vi "Figure Window.vi"(4 "Y scale label (amplitude (V))":string="amplitude (V)", 5 "Data name (samples)":string="samples", 6 "X scale label (time(s))":string="time (s)", 7 "Plot name (sampled signal)":string="Sampled signal", 11 "data qeue":refnum<queue>) -> ()   [LabVIEW 2020]
uses:
  <vilib>/Utility/error.llb/Error Cluster From Error Code.vi
  <vilib>/ErrorRing/Error Ring.xnode
  external libraries/varilib/varilib.lvlib
panel:
  out "external called for stop":bool
  out "title":string
  in  "Keep opened":bool=TRUE
  out "XY Graph":cluster{dbl[], dbl[]}(graph)
  in  "rectangle zoom":bool
  in  "zoom out":bool
  in  "y zoom":bool
  in  "x zoom":bool
  out "gui_elements":refnum<vi>[](array[refnum])
  in  "cancel":bool
  in  "export to excell":bool
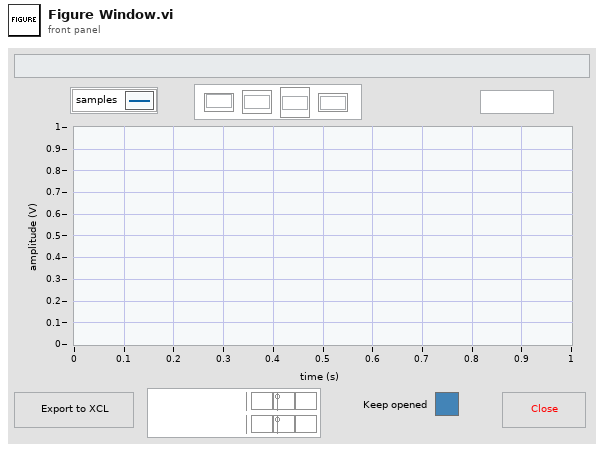
[diagram p1: front panel]
types:
  T1 = typedef "LVRectTypeDef.ctl" = cluster{"Left":i16, "Top":i16, "Right":i16, "Bottom":i16}
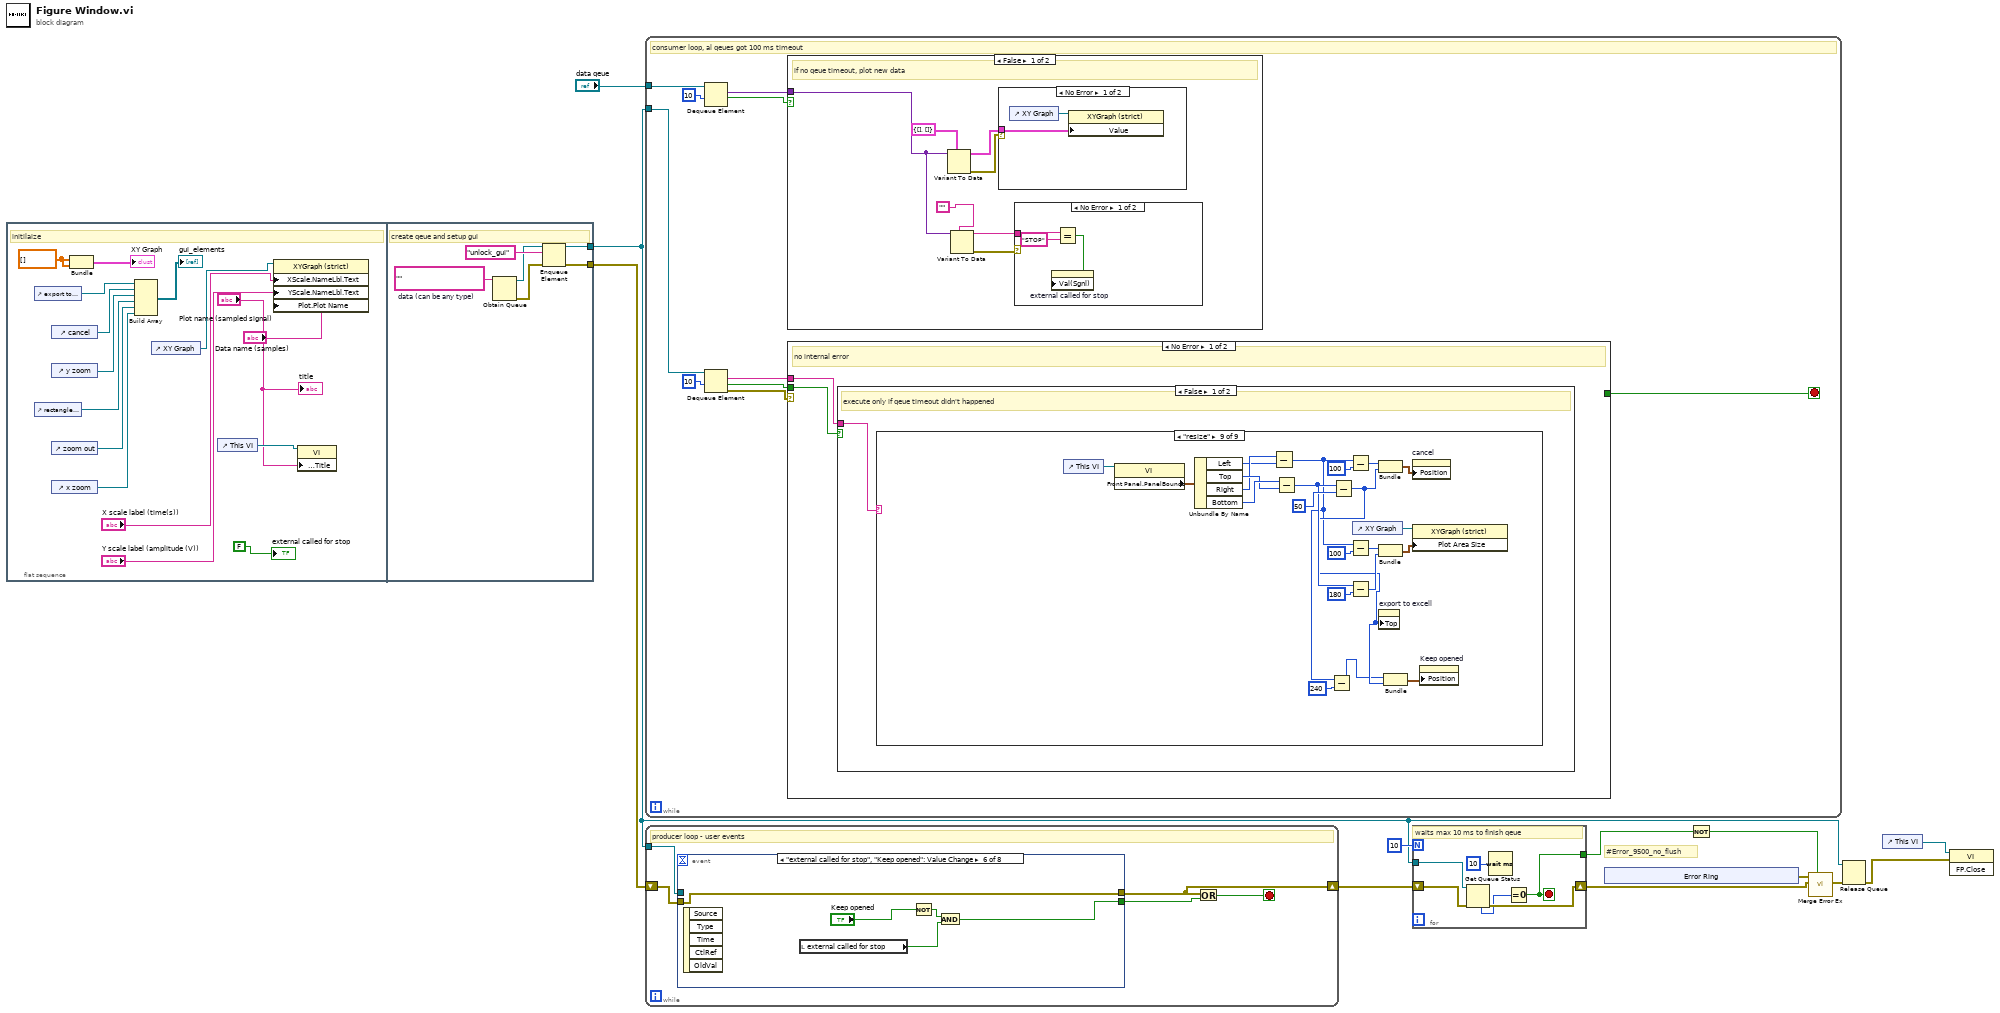
[diagram p0: block diagram]
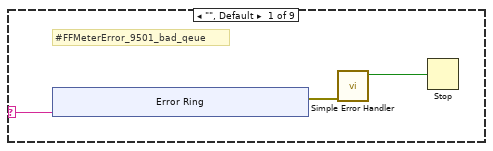
[diagram p5: hidden frame]
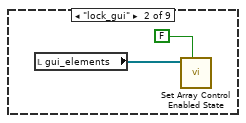
[diagram p6: hidden frame]
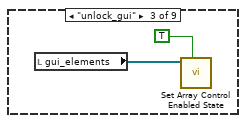
[diagram p7: hidden frame]
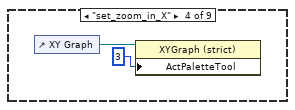
[diagram p8: hidden frame]
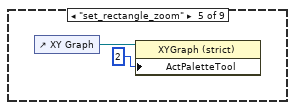
[diagram p9: hidden frame]
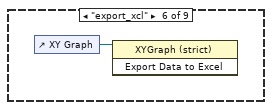
[diagram p10: hidden frame]
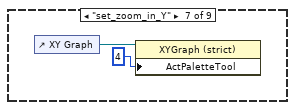
[diagram p11: hidden frame]
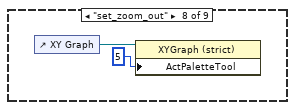
[diagram p12: hidden frame]
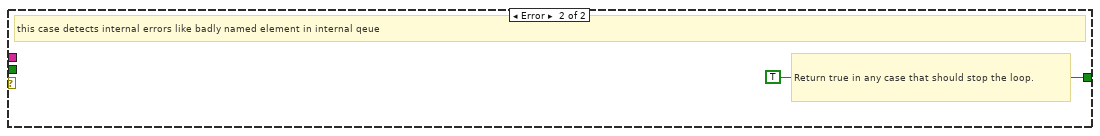
[diagram p14: hidden frame]
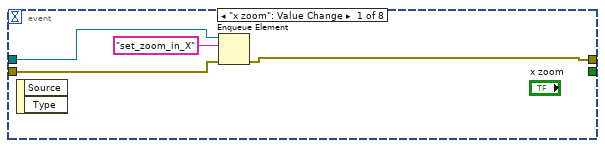
[diagram p15: hidden frame]
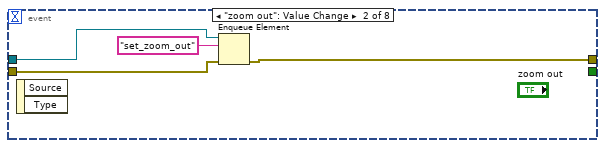
[diagram p16: hidden frame]
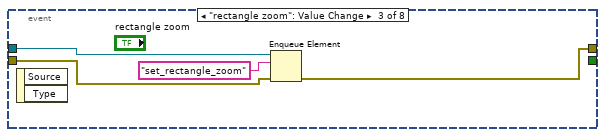
[diagram p17: hidden frame]
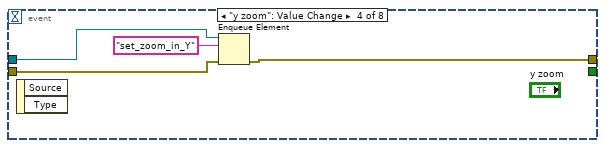
[diagram p18: hidden frame]
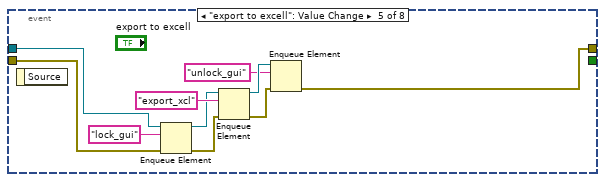
[diagram p19: hidden frame]
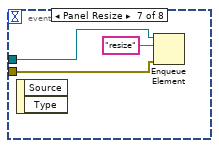
[diagram p20: hidden frame]
diagram:
  # "#Error_9500_no_flush"
  n1 = flat-sequence {
    tunnel: [w33] -> w5
    tunnel: [w31] -> w4
    frame #0 {
      w20 = dbl[] []
      # "initilaize"
      n2 = control-ref of="export to excell"() -> (w28:refnum<vi>)
      n3 = control-ref of="rectangle zoom"() -> (w24:refnum<vi>)
      n4 = control-ref of="cancel"() -> (w27:refnum<vi>)
      n5 = control-ref of="y zoom"() -> (w25:refnum<vi>)
      n6 = control-ref of="zoom out"() -> (w23:refnum<vi>)
      n7 = control-ref of="x zoom"() -> (w22:refnum<vi>)
      n8 = Bundle(w20, w20) -> (→"XY Graph":cluster{dbl[], dbl[]})  [unwired: 1 in]
      n9 = Build Array(w28, w27, w25, w24, w23, w22) -> (→"gui_elements":refnum<vi>[])
      n10 = control-ref of="XY Graph"() -> (w19:refnum<vi>)
      n11 = control-ref of="This VI"() -> (w16:refnum<vi>)
      n12 = property class="XYGraph (strict)"(reference=w19, "XScale.NameLbl.Text"="X scale label (time(s))", "YScale.NameLbl.Text"="Y scale label (amplitude (V))", "Plot.Plot Name"="Data name (samples)") -> ()  [unwired: 1 in, 2 out]
      n13 = property class="VI"(reference=w16, "Front Panel.Title"="Plot name (sampled signal)") -> ()  [unwired: 1 in, 2 out]
      "title" <- "Plot name (sampled signal)"
      "external called for stop" <- FALSE ("external called for stop")
    }
    frame #1 {
      w32 = ""  # data (can be any type)
      # "create qeue and setup gui"
      n14 = Obtain Queue(element data type=w32) -> (queue out=w30:refnum<queue>, error out=w29:errorcluster)  [unwired: 4 in, 1 out]
      n15 = Enqueue Element(queue=w30, element="unlock_gui", error in (no error)=w29) -> (queue out=w33:refnum<queue>, error out=w31:errorcluster)  [unwired: 1 in, 1 out]
    }
  }
  n16 = while {
    tunnel: w5 -> [w44]
    tunnel: "data qeue" -> [w37]
    stop <- w41 stop-if-true
    # "consumer loop, al qeues got 100 ms timeout"
    n17 = Dequeue Element(queue=w37, timeout in ms (-1)=10) -> (element=w38:variant, timed out?=w39:bool)  [unwired: 1 in, 2 out]
    n18 = Dequeue Element(queue=w44, timeout in ms (-1)=10) -> (element=w42:string, timed out?=w35:bool, error out=w43:errorcluster)  [unwired: 1 in, 1 out]
    n19 = case shown="False" w39 {
      tunnel: w38 -> [w47 _]
      frame False {
        # "if no qeue timeout, plot new data"
        n20 = Variant To Data(type=cluster{dbl[], dbl[]} {[], []} ("output cluster"), Variant=w47) -> (data=w50:cluster{dbl[], dbl[]}, error out=w49:errorcluster)  [unwired: 1 in]
        n21 = Variant To Data(type="", Variant=w47) -> (data=w45:string, error out=w46:errorcluster)  [unwired: 1 in]
        n22 = case shown="No Error" w49 {
          tunnel: w50 -> [w56 _]
          frame No Error {
            n23 = control-ref of="XY Graph"() -> (w55:refnum<vi>)
            n24 = property class="XYGraph (strict)"(reference=w55, "Value"=w56) -> ()  [unwired: 1 in, 2 out]
          }
          frame Error {
          }
        }
        n25 = case shown="No Error" w46 {
          tunnel: w45 -> [w54 _]
          frame No Error {
            n26 = Equal?(x=w54, y="STOP") -> (x = y?=w52:bool)
            n27 = property on="external called for stop" class="Bool (strict)"("Val(Sgnl)"=w52) -> ()  [unwired: 2 in, 2 out]
          }
          frame Error {
          }
        }
      }
      frame True {
      }
    }
    n28 = case shown="No Error" w43 {
      tunnel: w42 -> [w58 _]
      tunnel: [_ TRUE] -> w41
      tunnel: w35 -> [w57 _]
      frame No Error {
        # "no internal error"
        n29 = case shown="False" w57 {
          tunnel: w58 -> [w59 _]
          frame False {
            # "execute only if qeue timeout didn't happened"
            n30 = case shown="\"resize\"" w59 {
              selector: w59 -> [w60 _ _ _ _ _ _ _ _]
              frame "", Default {
                # "#FFMeterError_9501_bad_qeue"
                n31 = xnode "Error Ring"("parameter 0"=w60) -> ("error out"=w62:errorcluster)
                n32 = call <vilib>:"Simple Error Handler.vi"("error in (no error)"=w62) -> ("error?"=w61:bool)  [unwired: 4 in, 4 out]
                n33 = Stop(stop? (T)=w61) -> ()
              }
              frame "lock_gui" {
                n34 = local read "gui_elements"() -> (w71:refnum<vi>[])
                n35 = call "Set Array Control Enabled State.vi"("enabled (T)"=FALSE, "reference array in"=w71) -> ()  [unwired: 8 in, 2 out]
              }
              frame "unlock_gui" {
                n36 = local read "gui_elements"() -> (w73:refnum<vi>[])
                n37 = call "Set Array Control Enabled State.vi"("enabled (T)"=TRUE, "reference array in"=w73) -> ()  [unwired: 8 in, 2 out]
              }
              frame "set_zoom_in_X" {
                n38 = control-ref of="XY Graph"() -> (w74:refnum<vi>)
                n39 = property class="XYGraph (strict)"(reference=w74, "ActPaletteTool"=3 ("Palette:Active Tool")) -> ()  [unwired: 1 in, 2 out]
              }
              frame "set_rectangle_zoom" {
                n40 = control-ref of="XY Graph"() -> (w76:refnum<vi>)
                n41 = property class="XYGraph (strict)"(reference=w76, "ActPaletteTool"=2 ("Palette:Active Tool")) -> ()  [unwired: 1 in, 2 out]
              }
              frame "export_xcl" {
                n42 = control-ref of="XY Graph"() -> (w78:refnum<vi>)
                n43 = invoke class="XYGraph (strict)" method="Export Data to Excel"(reference=w78) -> ()  [unwired: 2 in, 3 out]
              }
              frame "set_zoom_in_Y" {
                n44 = control-ref of="XY Graph"() -> (w79:refnum<vi>)
                n45 = property class="XYGraph (strict)"(reference=w79, "ActPaletteTool"=4 ("Palette:Active Tool")) -> ()  [unwired: 1 in, 2 out]
              }
              frame "set_zoom_out" {
                n46 = control-ref of="XY Graph"() -> (w81:refnum<vi>)
                n47 = property class="XYGraph (strict)"(reference=w81, "ActPaletteTool"=5 ("Palette:Active Tool")) -> ()  [unwired: 1 in, 2 out]
              }
              frame "resize" {
                n48 = control-ref of="This VI"() -> (w90:refnum<vi>)
                n49 = property class="VI"(reference=w90) -> ("Front Panel.PanelBounds"=w91:T1)  [unwired: 1 in, 2 out]
                n50 = Unbundle By Name(w91) -> ("Left"=w92:i16, "Top"=w95:i16, "Right"=w93:i16, "Bottom"=w96:i16)
                n51 = Subtract(x=w93, y=w92) -> (x-y=w83:i16)
                n52 = Subtract(x=w96, y=w95) -> (x-y=w94:i16)
                n53 = Subtract(x=w83, y=i16 240) -> (x-y=w84:i16)
                n54 = Subtract(x=w94, y=i16 50) -> (x-y=w86:i16)
                n55 = Subtract(x=w83, y=i16 100) -> (x-y=w103:i16)
                n56 = Subtract(x=w83, y=i16 100) -> (x-y=w98:i16)
                n57 = Subtract(x=w94, y=i16 180) -> (x-y=w97:i16)
                n58 = control-ref of="XY Graph"() -> (w88:refnum<vi>)
                n59 = Bundle(w103, w86) -> (w104:cluster{i16, i16})  [unwired: 1 in]
                n60 = Bundle(w98, w97) -> (w89:cluster{i16, i16})  [unwired: 1 in]
                n61 = property on="export to excell" class="Bool"("Top"=w86) -> ()  [unwired: 2 in, 2 out]
                n62 = Bundle(w84, w86) -> (w87:cluster{i16, i16})  [unwired: 1 in]
                n63 = property on="cancel" class="Bool"("Position"=w104) -> ()  [unwired: 2 in, 2 out]
                n64 = property class="XYGraph (strict)"(reference=w88, "Plot Area Size"=w89) -> ()  [unwired: 1 in, 2 out]
                n65 = property on="Keep opened" class="Bool (strict)"("Position"=w87) -> ()  [unwired: 2 in, 2 out]
              }
            }
          }
          frame True {
          }
        }
      }
      frame Error {
        # "Return true in any case that should stop the loop."
        # "this case detects internal errors like badly named element in internal qeue"
      }
    }
  }
  n66 = while {
    shift-right: [w106] -> w8
    shift-left: w4 -> [w109]
    tunnel: w5 -> [w110]
    stop <- w107 stop-if-true
    # "producer loop - user events"
    n67 = event shown="[5] \"external called for stop\", \"Keep opened\": Value Change" {
      selector: _ -> [_ _ _ _ _ _ _ _]
      dyn-events: _ -> [_ _ _ _ _ _ _ _]
      timeout: _ -> [_ _ _ _ _ _ _ _]
      tunnel: w110 -> [w111 w115 w119 w123 w134 _ w143 _]
      tunnel: w109 -> [w112 w116 w120 w124 w133 w141 w142 w146]
      tunnel: [w113 w117 w121 w125 w127 w141 _ w146] -> w106
      tunnel: [_ _ _ _ _ w139 _ TRUE ("cancel")] -> w108
      event "x zoom": Value Change {
        n68 = event-data() -> ()  [unwired: 1 in, 2 out]
        n69 = Enqueue Element(queue=w111, element="set_zoom_in_X", error in (no error)=w112) -> (error out=w113:errorcluster)  [unwired: 1 in, 2 out]
      }
      event "zoom out": Value Change {
        n70 = event-data() -> ()  [unwired: 1 in, 2 out]
        n71 = Enqueue Element(queue=w115, element="set_zoom_out", error in (no error)=w116) -> (error out=w117:errorcluster)  [unwired: 1 in, 2 out]
      }
      event "rectangle zoom": Value Change {
        n72 = event-data() -> ()  [unwired: 1 in, 2 out]
        n73 = Enqueue Element(queue=w119, element="set_rectangle_zoom", error in (no error)=w120) -> (error out=w121:errorcluster)  [unwired: 1 in, 2 out]
      }
      event "y zoom": Value Change {
        n74 = event-data() -> ()  [unwired: 1 in, 2 out]
        n75 = Enqueue Element(queue=w123, element="set_zoom_in_Y", error in (no error)=w124) -> (error out=w125:errorcluster)  [unwired: 1 in, 2 out]
      }
      event "export to excell": Value Change {
        n76 = event-data() -> ()  [unwired: 1 in, 1 out]
        n77 = Enqueue Element(queue=w134, element="lock_gui", error in (no error)=w133) -> (queue out=w131:refnum<queue>, error out=w132:errorcluster)  [unwired: 1 in, 1 out]
        n78 = Enqueue Element(queue=w131, element="export_xcl", error in (no error)=w132) -> (queue out=w130:refnum<queue>, error out=w129:errorcluster)  [unwired: 1 in, 1 out]
        n79 = Enqueue Element(queue=w130, element="unlock_gui", error in (no error)=w129) -> (error out=w127:errorcluster)  [unwired: 1 in, 2 out]
      }
      event "external called for stop", "Keep opened": Value Change {
        n80 = event-data() -> ()  [unwired: 1 in, 5 out]
        n81 = local read "external called for stop"() -> (w140:bool)
        n82 = Not(x="Keep opened") -> (.not. x?=w138:bool)
        n83 = And(x=w138, y=w140) -> (x .and. y?=w139:bool)
      }
      event Panel Resize {
        n84 = event-data() -> ()  [unwired: 1 in, 2 out]
        n85 = Enqueue Element(queue=w143, element="resize", error in (no error)=w142) -> ()  [unwired: 1 in, 3 out]
      }
      event "cancel": Value Change; Panel Close {
        n86 = event-data() -> ()  [unwired: 1 in, 2 out]
      }
    }
    n87 = Or(x=w106, y=w108) -> (x .or. y?=w107:bool)
  }
  n88 = for {
    N: 10 -> [_]
    tunnel: w5 -> [w152]
    shift-right: [w150] -> w9
    shift-left: w8 -> [w151]
    tunnel: [w147] -> w6
    stop <- w147 stop-if-true
    # "waits max 10 ms to finish qeue"
    n89 = Get Queue Status(queue=w152, error in (no error)=w151) -> (error out=w150:errorcluster, # elements in queue=w148:i32)  [unwired: 1 in, 6 out]
    n90 = Wait (ms)(milliseconds to wait=u32 10) -> ()  [unwired: 1 out]
    n91 = Equal To 0?(x=w148) -> (x = 0?=w147:bool)
  }
  n92 = xnode "Error Ring"() -> ("error out"=w10:errorcluster)
  n93 = Not(x=w6) -> (.not. x?=w11:bool)
  n94 = call "Merge Error Ex.vi"("Is error? (False)"=w11, "main error in (no error)"=w9, "second error in"=w10) -> ("error out"=w7:errorcluster)  [unwired: 8 in]
  n95 = Release Queue(queue=w5, error in (no error)=w7) -> (error out=w2:errorcluster)  [unwired: 1 in, 2 out]
  n96 = control-ref of="This VI"() -> (w3:refnum<vi>)
  n97 = invoke class="VI" method="FP.Close"(reference=w3, error in=w2) -> ()  [unwired: 1 in, 3 out]
